vi "Set X Maximum.vi"(9 "output cluster":T1, 11 "Display Size":T2(ring)) -> ()   [LabVIEW 2014]
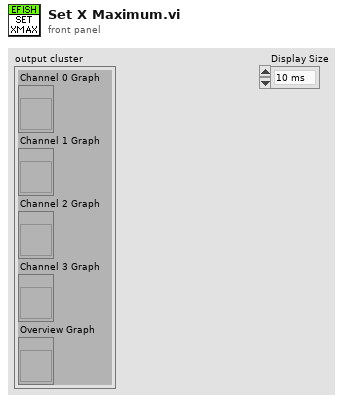
[diagram p1: front panel]
types:
  T1 = cluster{"Channel 0 Graph":refnum<vi>, "Channel 1 Graph":refnum<vi>, "Channel 2 Graph":refnum<vi>, "Channel 3 Graph":refnum<vi>, "Overview Graph":refnum<vi>}
  T2 = enum16{"10 ms", "100 ms", "1 Second", "10 sec", "30 sec"}
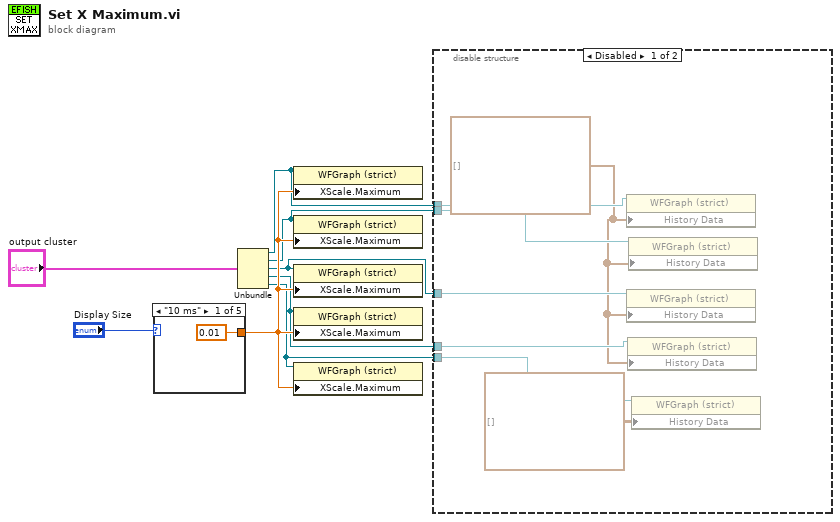
[diagram p0: block diagram]
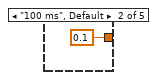
[diagram p3: hidden frame]
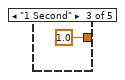
[diagram p4: hidden frame]
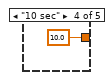
[diagram p5: hidden frame]
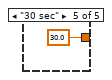
[diagram p6: hidden frame]
diagram:
  n1 = case shown="\"10 ms\"" "Display Size" {
    tunnel: [0.01 0.1 1.0 10.0 30.0] -> w8
    frame "10 ms" {
    }
    frame "100 ms", Default {
    }
    frame "1 Second" {
    }
    frame "10 sec" {
    }
    frame "30 sec" {
    }
  }
  n2 = Unbundle("output cluster") -> ("Channel 0 Graph"=w6:refnum<vi>, "Channel 1 Graph"=w5:refnum<vi>, "Channel 2 Graph"=w4:refnum<vi>, "Channel 3 Graph"=w3:refnum<vi>, "Overview Graph"=w2:refnum<vi>)
  n3 = property on="Property Node" class="WFGraph (strict)"(reference=w6, "XScale.Maximum"=w8) -> ()  [unwired: 1 in, 2 out]
  n4 = property on="Property Node" class="WFGraph (strict)"(reference=w5, "XScale.Maximum"=w8) -> ()  [unwired: 1 in, 2 out]
  n5 = property on="Property Node" class="WFGraph (strict)"(reference=w4, "XScale.Maximum"=w8) -> ()  [unwired: 1 in, 2 out]
  n6 = property on="Property Node" class="WFGraph (strict)"(reference=w3, "XScale.Maximum"=w8) -> ()  [unwired: 1 in, 2 out]
  n7 = property on="Property Node" class="WFGraph (strict)"(reference=w2, "XScale.Maximum"=w8) -> ()  [unwired: 1 in, 2 out]
  n8 = disable-structure shown="Disabled" {
    disable-tunnel: w6 -> [w20 _]
    disable-tunnel: w5 -> [w19 _]
    disable-tunnel: w4 -> [w18 _]
    disable-tunnel: w3 -> [w17 _]
    disable-tunnel: w2 -> [w16 _]
    frame Disabled {
      w15 = waveform(dbl)[] [] ("History Data")
      n9 = property on="Property Node" class="WFGraph (strict)"(reference=w20, "History Data"=w15) -> ()  [unwired: 1 in, 2 out]
      n10 = property on="Property Node" class="WFGraph (strict)"(reference=w18, "History Data"=w15) -> ()  [unwired: 1 in, 2 out]
      n11 = property on="Property Node" class="WFGraph (strict)"(reference=w17, "History Data"=w15) -> ()  [unwired: 1 in, 2 out]
      n12 = property on="Property Node" class="WFGraph (strict)"(reference=w19, "History Data"=w15) -> ()  [unwired: 1 in, 2 out]
      n13 = property on="Property Node" class="WFGraph (strict)"(reference=w16, "History Data"=waveform(dbl)[][] []) -> ()  [unwired: 1 in, 2 out]
    }
    frame Enabled {
    }
  }
